vi "Gen - Get Module Name.vi"(8 "error in (no error)":errorcluster, 11 "VI in":refnum<vi>) -> (0 "error out":errorcluster, 3 "result string":string)   [LabVIEW 2020]
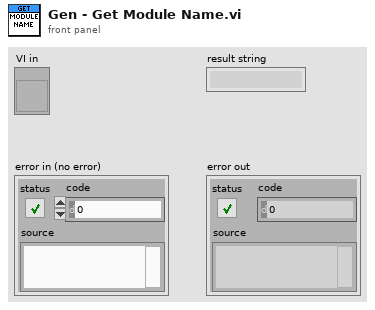
[diagram p1: front panel]
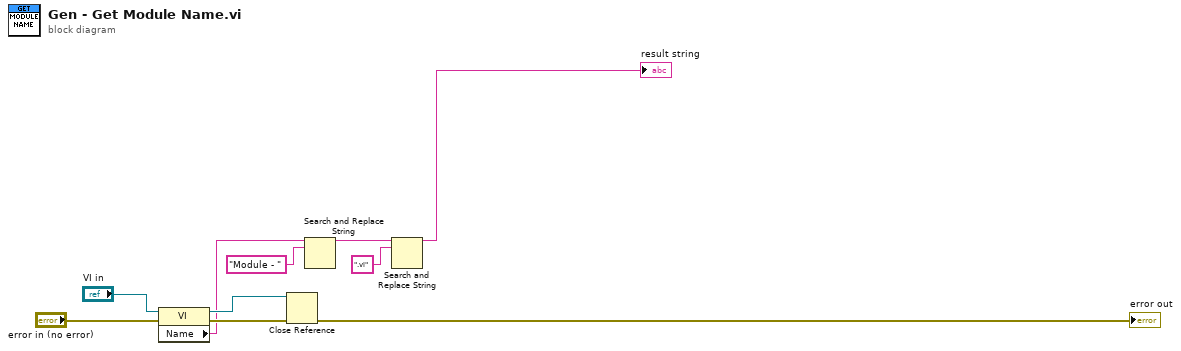
[diagram p0: block diagram]
diagram:
  n1 = property class="VI"(reference="VI in", error in="error in (no error)") -> (reference out=w7:refnum<vi>, error out=w6:errorcluster, "Name"=w2:string)
  n2 = Close Reference(reference=w7, error in (no error)=w6) -> (error out=→"error out":errorcluster)
  n3 = Search and Replace String(input string=w2, search string="Module - ") -> (result string=w5:string)  [unwired: 6 in, 3 out]
  n4 = Search and Replace String(input string=w5, search string=".vi") -> (result string=→"result string":string)  [unwired: 6 in, 3 out]
